vi "Requests.vi"(8 "error in (no error)":errorcluster, 9 "write enable":bool=TRUE, 11 "MB_TCP in":refnum<class "MB_TCP.lvclass">) -> (0 "error out":errorcluster, 3 "MB_TCP out":refnum<class "MB_TCP.lvclass">)   [LabVIEW 2019, in "MB_TCP.lvclass"]
uses:
  MB_TCP.lvclass
  ICPCON Registers/ICPCON Registers.lvlib
  Timer Delay/Timers.lvlib
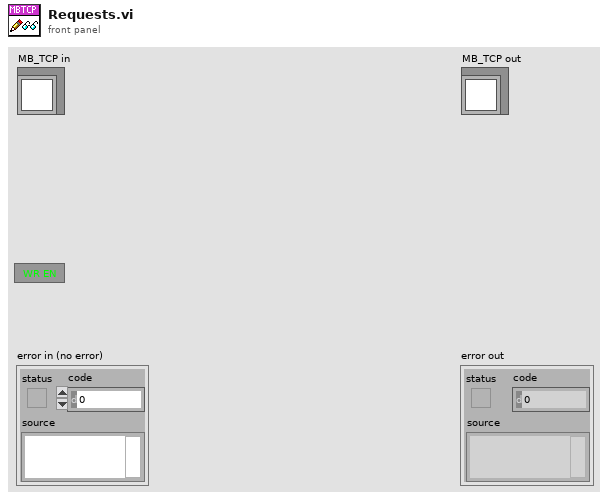
[diagram p1: front panel]
types:
  T1 = typedef "ICPCON Registers.lvlib/ICPCON Data.ctl" = cluster{"UTF":refnum<data-value>, "DI":refnum<data-value>, "DW":refnum<data-value>, "DO":refnum<data-value>, "IR":refnum<data-value>, "WR":refnum<data-value>, "OR":refnum<data-value>, "Initialised":bool}
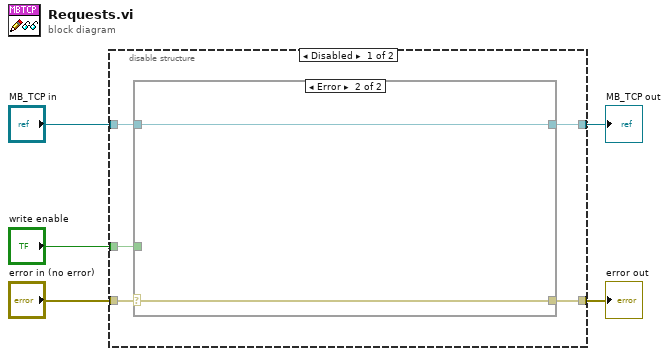
[diagram p0: block diagram]
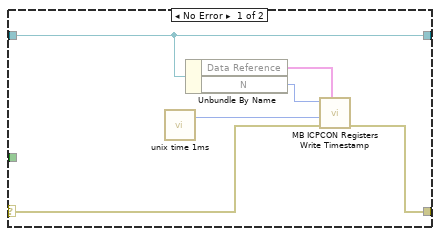
[diagram p2: hidden frame]
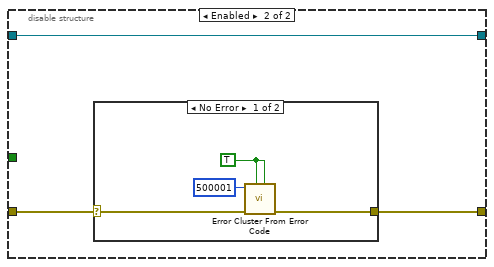
[diagram p3: hidden frame]
diagram:
  n1 = disable-structure shown="Disabled" {
    disable-tunnel: "error in (no error)" -> [w10 w19]
    disable-tunnel: [w9 w20] -> w4
    disable-tunnel: "MB_TCP in" -> [w8 w21]
    disable-tunnel: [w7 w21] -> w1
    disable-tunnel: "write enable" -> [w6 _]
    frame Disabled {
      n2 = case shown="Error" w10 {
        selector: w10 -> [w13 w18]
        tunnel: [w14 w18] -> w9
        tunnel: [w16 w17] -> w7
        tunnel: w8 -> [w16 w17]
        tunnel: w6 -> [_ _]
        frame No Error {
          n3 = call "unix time 1ms.vi"() -> ("unix time (ms)"=w11:u64)  [unwired: 2 in, 1 out]
          n4 = Unbundle By Name(w16) -> ("Data Reference"=w15:T1, "N"=w12:i32)
          n5 = call "MB ICPCON Registers Write Timestamp.vi"("Data Reference"=w15, "error in (no error)"=w13, "UTF"=w11, "N"=w12) -> ("error out"=w14:errorcluster)  [unwired: 7 in]
        }
        frame Error {
        }
      }
    }
    frame Enabled {
      n6 = case shown="No Error" w19 {
        selector: w19 -> [w22 w26]
        tunnel: [w23 w26] -> w20
        frame No Error {
          w24 = TRUE ("show call chain? (False)")
          n7 = call <vilib>:"Error Cluster From Error Code.vi"("is warning? (False)"=w24, "show call chain? (False)"=w24, "error in (no error)"=w22, "error code (0)"=500001) -> ("error out"=w23:errorcluster)  [unwired: 5 in]
        }
        frame Error {
        }
      }
    }
  }
  "error out" <- w4
  "MB_TCP out" <- w1
